vi "Msg Not Implemented --error.vi"() -> (2 "Error":errorcluster)   [LabVIEW 2020, in "jettl.lvlib" / "Error.lvlib"]
uses:
  Error.lvlib
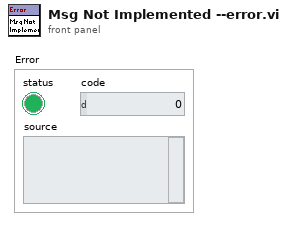
[diagram p1: front panel]
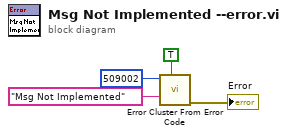
[diagram p0: block diagram]
diagram:
  n1 = call <vilib>:"Error Cluster From Error Code.vi"("show call chain? (False)"=TRUE, "error message (\"\")"="Msg Not Implemented" ("error message (\"\")"), "error code (0)"=509002) -> ("error out"=→"Error":errorcluster)  [unwired: 6 in]
